vi "S2C_PCIe7841_Proc_AnalogWriteLocal.vi"(8 "Error In":errorcluster, 9 "ExeRef":refnum<vi>, 11 "Q-Ref":refnum<queue>) -> (0 "Error Out":errorcluster, 3 "Command":string)   [LabVIEW 2015]
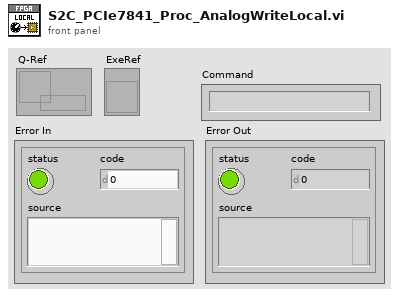
[diagram p1: front panel]
types:
  T1 = cluster{"AO0":dbl, "AO0_Send":bool, "AO1":dbl, "AO1_Send":bool, "AO2":dbl, "AO2_Send":bool, "AO3":dbl, "AO3_Send":bool, "AO4":dbl, "AO4_Send":bool, "AO5":dbl, "AO5_Send":bool, "AO6":dbl, "AO6_Send":bool, "AO7":dbl, "AO7_Send":bool, "P6C1Exe":bool}
  T2 = cluster{"Caller-Q":refnum<queue>, "Command":string, "Return":string, "Data":variant, "Timeout":dbl}
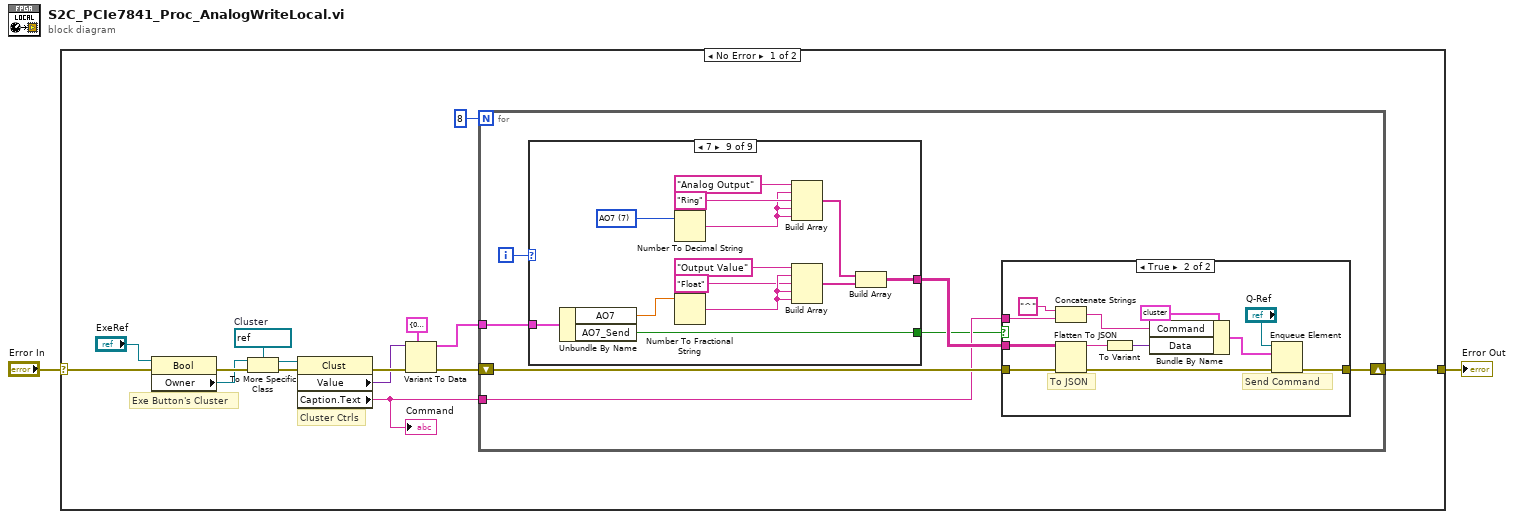
[diagram p0: block diagram]
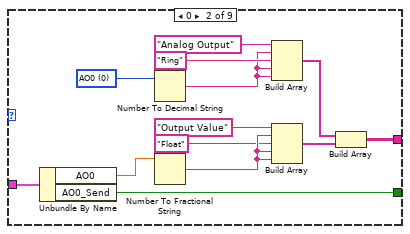
[diagram p4: hidden frame]
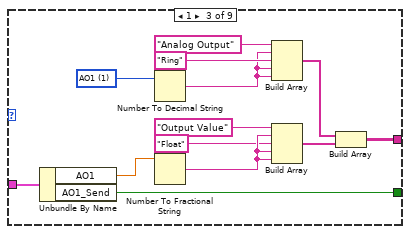
[diagram p5: hidden frame]
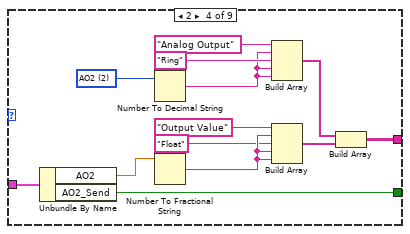
[diagram p6: hidden frame]
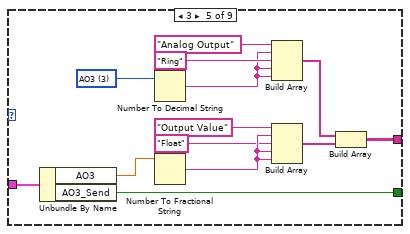
[diagram p7: hidden frame]
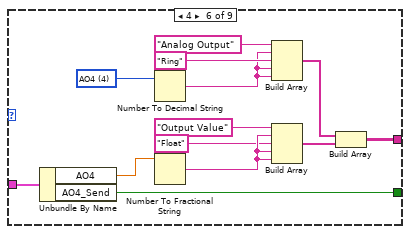
[diagram p8: hidden frame]
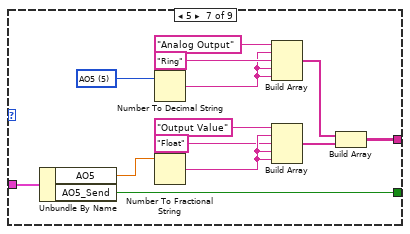
[diagram p9: hidden frame]
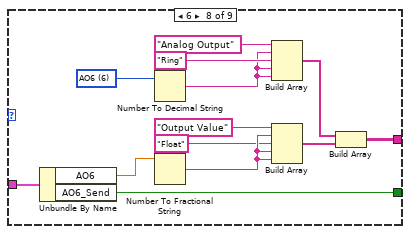
[diagram p10: hidden frame]
diagram:
  n1 = case shown="No Error" "Error In" {
    selector: "Error In" -> [w11 w142]
    tunnel: [w4 w142] -> w1
    frame No Error {
      w14 = refnum<vi> refnum  # Cluster
      # "Cluster Ctrls"
      # "Exe Button's Cluster"
      n2 = property class="Bool"(reference="ExeRef", error in=w11) -> (error out=w16:errorcluster, "Owner"=w15:refnum<vi>)  [unwired: 1 out]
      n3 = To More Specific Class(target class=w14, reference=w15, error in=w16) -> (specific class reference=w12:refnum<vi>, error out=w13:errorcluster)
      n4 = property class="Clust"(reference=w12, error in=w13) -> (error out=w10:errorcluster, "Value"=w9:variant, "Caption.Text"=w3:string)  [unwired: 1 out]
      "Command" <- w3
      n5 = Variant To Data(error in=w10, type=T1 {"AO0"=0.0, "AO0_Send"=FALSE, "AO1"=0.0, "AO1_Send"=FALSE, "AO2"=0.0, "AO2_Send"=FALSE, "AO3"=0.0, "AO3_Send"=FALSE, "AO4"=0.0, "AO4_Send"=FALSE, "AO5"=0.0, "AO5_Send"=FALSE, "AO6"=0.0, "AO6_Send"=FALSE, "AO7"=0.0, "AO7_Send"=FALSE, "P6C1Exe"=FALSE} ("Analog Output"), Variant=w9) -> (data=w7:T1, error out=w5:errorcluster)
      n6 = for {
        N: 8 -> [_]
        tunnel: w7 -> [w24]
        shift-right: [w21] -> w4
        shift-left: w5 -> [w22]
        tunnel: w3 -> [w19]
        i -> [w23]
        n7 = case shown="7" w23 {
          tunnel: w24 -> [_ w46 w59 w72 w85 w98 w111 w124 w137]
          tunnel: [_ w39 w52 w65 w78 w91 w104 w117 w130] -> w18
          tunnel: [_ w38 w51 w64 w77 w90 w103 w116 w129] -> w20
          frame -1, Default {
          }
          frame 0 {
            w42 = u16 0 items=["AO0", "AO1", "AO2", "AO3", "AO4", "AO5", "AO6", "AO7"] ("Analog Output")
            n8 = Unbundle By Name(w46) -> ("AO0"=w47:dbl, "AO0_Send"=w39:bool)
            n9 = Number To Decimal String(number=w42) -> (decimal integer string=w43:string)  [unwired: 1 in]
            n10 = Number To Fractional String(number=w47) -> (F-format string=w50:string)  [unwired: 3 in]
            n11 = Build Array("Analog Output" ("element"), w43, "Ring", w43, w43) -> (w41:string[])
            n12 = Build Array("Output Value" ("element"), w50, "Float", w50, w50) -> (w40:string[])
            n13 = Build Array(w41, w40) -> (w38:string[][])
          }
          frame 1 {
            w55 = u16 1 items=["AO0", "AO1", "AO2", "AO3", "AO4", "AO5", "AO6", "AO7"] ("Analog Output")
            n14 = Unbundle By Name(w59) -> ("AO1"=w60:dbl, "AO1_Send"=w52:bool)
            n15 = Number To Decimal String(number=w55) -> (decimal integer string=w56:string)  [unwired: 1 in]
            n16 = Number To Fractional String(number=w60) -> (F-format string=w63:string)  [unwired: 3 in]
            n17 = Build Array("Analog Output" ("element"), w56, "Ring", w56, w56) -> (w54:string[])
            n18 = Build Array("Output Value" ("element"), w63, "Float", w63, w63) -> (w53:string[])
            n19 = Build Array(w54, w53) -> (w51:string[][])
          }
          frame 2 {
            w68 = u16 2 items=["AO0", "AO1", "AO2", "AO3", "AO4", "AO5", "AO6", "AO7"] ("Analog Output")
            n20 = Unbundle By Name(w72) -> ("AO2"=w73:dbl, "AO2_Send"=w65:bool)
            n21 = Number To Decimal String(number=w68) -> (decimal integer string=w69:string)  [unwired: 1 in]
            n22 = Number To Fractional String(number=w73) -> (F-format string=w76:string)  [unwired: 3 in]
            n23 = Build Array("Analog Output" ("element"), w69, "Ring", w69, w69) -> (w67:string[])
            n24 = Build Array("Output Value" ("element"), w76, "Float", w76, w76) -> (w66:string[])
            n25 = Build Array(w67, w66) -> (w64:string[][])
          }
          frame 3 {
            w81 = u16 3 items=["AO0", "AO1", "AO2", "AO3", "AO4", "AO5", "AO6", "AO7"] ("Analog Output")
            n26 = Unbundle By Name(w85) -> ("AO3"=w86:dbl, "AO3_Send"=w78:bool)
            n27 = Number To Decimal String(number=w81) -> (decimal integer string=w82:string)  [unwired: 1 in]
            n28 = Number To Fractional String(number=w86) -> (F-format string=w89:string)  [unwired: 3 in]
            n29 = Build Array("Analog Output" ("element"), w82, "Ring", w82, w82) -> (w80:string[])
            n30 = Build Array("Output Value" ("element"), w89, "Float", w89, w89) -> (w79:string[])
            n31 = Build Array(w80, w79) -> (w77:string[][])
          }
          frame 4 {
            w94 = u16 4 items=["AO0", "AO1", "AO2", "AO3", "AO4", "AO5", "AO6", "AO7"] ("Analog Output")
            n32 = Unbundle By Name(w98) -> ("AO4"=w99:dbl, "AO4_Send"=w91:bool)
            n33 = Number To Decimal String(number=w94) -> (decimal integer string=w95:string)  [unwired: 1 in]
            n34 = Number To Fractional String(number=w99) -> (F-format string=w102:string)  [unwired: 3 in]
            n35 = Build Array("Analog Output" ("element"), w95, "Ring", w95, w95) -> (w93:string[])
            n36 = Build Array("Output Value" ("element"), w102, "Float", w102, w102) -> (w92:string[])
            n37 = Build Array(w93, w92) -> (w90:string[][])
          }
          frame 5 {
            w107 = u16 5 items=["AO0", "AO1", "AO2", "AO3", "AO4", "AO5", "AO6", "AO7"] ("Analog Output")
            n38 = Unbundle By Name(w111) -> ("AO5"=w112:dbl, "AO5_Send"=w104:bool)
            n39 = Number To Decimal String(number=w107) -> (decimal integer string=w108:string)  [unwired: 1 in]
            n40 = Number To Fractional String(number=w112) -> (F-format string=w115:string)  [unwired: 3 in]
            n41 = Build Array("Analog Output" ("element"), w108, "Ring", w108, w108) -> (w106:string[])
            n42 = Build Array("Output Value" ("element"), w115, "Float", w115, w115) -> (w105:string[])
            n43 = Build Array(w106, w105) -> (w103:string[][])
          }
          frame 6 {
            w120 = u16 6 items=["AO0", "AO1", "AO2", "AO3", "AO4", "AO5", "AO6", "AO7"] ("Analog Output")
            n44 = Unbundle By Name(w124) -> ("AO6"=w125:dbl, "AO6_Send"=w117:bool)
            n45 = Number To Decimal String(number=w120) -> (decimal integer string=w121:string)  [unwired: 1 in]
            n46 = Number To Fractional String(number=w125) -> (F-format string=w128:string)  [unwired: 3 in]
            n47 = Build Array("Analog Output" ("element"), w121, "Ring", w121, w121) -> (w119:string[])
            n48 = Build Array("Output Value" ("element"), w128, "Float", w128, w128) -> (w118:string[])
            n49 = Build Array(w119, w118) -> (w116:string[][])
          }
          frame 7 {
            w133 = u16 7 items=["AO0", "AO1", "AO2", "AO3", "AO4", "AO5", "AO6", "AO7"] ("Analog Output")
            n50 = Unbundle By Name(w137) -> ("AO7"=w138:dbl, "AO7_Send"=w130:bool)
            n51 = Number To Decimal String(number=w133) -> (decimal integer string=w134:string)  [unwired: 1 in]
            n52 = Number To Fractional String(number=w138) -> (F-format string=w141:string)  [unwired: 3 in]
            n53 = Build Array("Analog Output" ("element"), w134, "Ring", w134, w134) -> (w132:string[])
            n54 = Build Array("Output Value" ("element"), w141, "Float", w141, w141) -> (w131:string[])
            n55 = Build Array(w132, w131) -> (w129:string[][])
          }
        }
        n56 = case shown="True" w18 {
          tunnel: w22 -> [w25 w29]
          tunnel: [w25 w28] -> w21
          tunnel: w20 -> [_ w27]
          tunnel: w19 -> [_ w26]
          frame False {
          }
          frame True {
            # "Send Command"
            # "To JSON"
            n57 = Concatenate Strings("^" ("string"), w26) -> (w33:string)
            n58 = Flatten To JSON(anything=w27, error in (no error)=w29) -> (JSON string=w31:string, 11:w30:errorcluster)  [unwired: 1 in]
            n59 = To Variant(anything=w31) -> (Variant=w35:variant)
            n60 = Bundle By Name(cluster=T2 {"Caller-Q"=refnum, "Command"="", "Return"="None", "Data"=variant, "Timeout"=10.0} ("element"), "Command"=w33, "Data"=w35) -> (w36:T2)
            n61 = Enqueue Element(queue="Q-Ref", element=w36, error in (no error)=w30) -> (error out=w28:errorcluster)  [unwired: 1 in, 2 out]
          }
        }
      }
    }
    frame Error {
    }
  }
  "Error Out" <- w1
